vi "Target.vi"() -> ()   [LabVIEW 2013]
uses:
  <vilib>/Platform/TimedLoop/XDataNode/XDataNode.xnode
  <vilib>/Platform/TimedLoop/XDataNode/nitl_modes.ctl
  <vilib>/Platform/TimedLoop/XDataNode/XDNodeRunTimeDep.lvlib
  <vilib>/Platform/TimedLoop/XDataNode/wakeup.ctl
  <vilib>/Platform/TimedLoop/XDataNode/timing_clust.ctl
  <vilib>/rvi/DataTransferAndStorage/Container/XNode/niFpgaContainer.xnode
  <vilib>/rvi/Memory/Memory_Emulation/niFpgaMemoryFastEmulationDramWriteAndRequestData.vi
  <vilib>/rvi/Memory/Memory_Emulation/niFpgaMemoryEmulationDramWriteAndRequestData.vi
  <vilib>/rvi/Memory/Memory_Emulation/niFpgaMemoryEmulationDramRetrieveData.vi
  <vilib>/rvi/interface/RandomDataEmulation/nirviRandomDataFpgaReadWriteTemplate.vi
panel:
  out "I":i32
  out "D-0 2":u16
  out "Addr":u32
  in  "Непрерывно":bool
  out "Number of Elements to Write":u32
  in  "Чтение FIFO":bool
  out "Data":u16
  in  "Input Valid":bool=TRUE
  in  "Address":u32
  in  "Чтение DRAM":bool
  in  "Начальный адрес":u32
  in  "HOST":bool
  in  "D-0":u16
  in  "Запись в DRAM":bool
  in  "Стоп":bool
  in  "Requested Number of Elements":u32=1073152
  in  "2/2":i16=40
  in  "1/2":i16=20
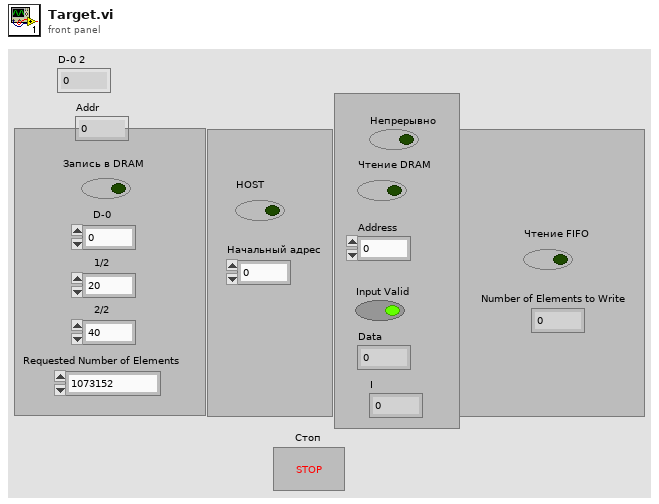
[diagram p1: front panel]
types:
  T1 = typedef "XDNodeRunTimeDep.lvlib/timing_clust.ctl" = cluster{"Expected End [f-1]":u64, "Actual End [f-1]":u64, "Finished Late? [f-1]":bool, "Expected End [i-1]":u64, "Actual End [i-1]":u64, "Finished Late? [i-1]":bool, "Expected Start [i]":u64, "Actual Start [i]":u64, "Expected Start [f]":u64, "Actual Start [f]":u64, "Source Name":string, "Structure Name":string, "Period":i64, "Deadline":i64, "Offset":i64, "Start":i64, "Priority":i32, "Timeout":i32, "Mode":T2, "Wakeup Reason":T3, "Error":errorcluster, "Source Type":string, "Secondary Source Type":string, "Global End Time":u64, "Global Start Time":u64, "Frame Duration":u64, "Iteration Duration":u64, "Assigned CPU":i32, "I/O Scan Engine Mode":u32}
  T2 = typedef "XDNodeRunTimeDep.lvlib/nitl_modes.ctl" = enum32{"No Change", "Process missed periods, maintain original phase", "Discard missed periods, maintain original phase", "Process missed periods, ignore original phase", "Discard missed periods, ignore original phase"}
  T3 = typedef "XDNodeRunTimeDep.lvlib/wakeup.ctl" = enum32{"Normal", "Aborted", "Asynchronous wakeup", "Timing source error", "Timed loop error", "Timeout"}
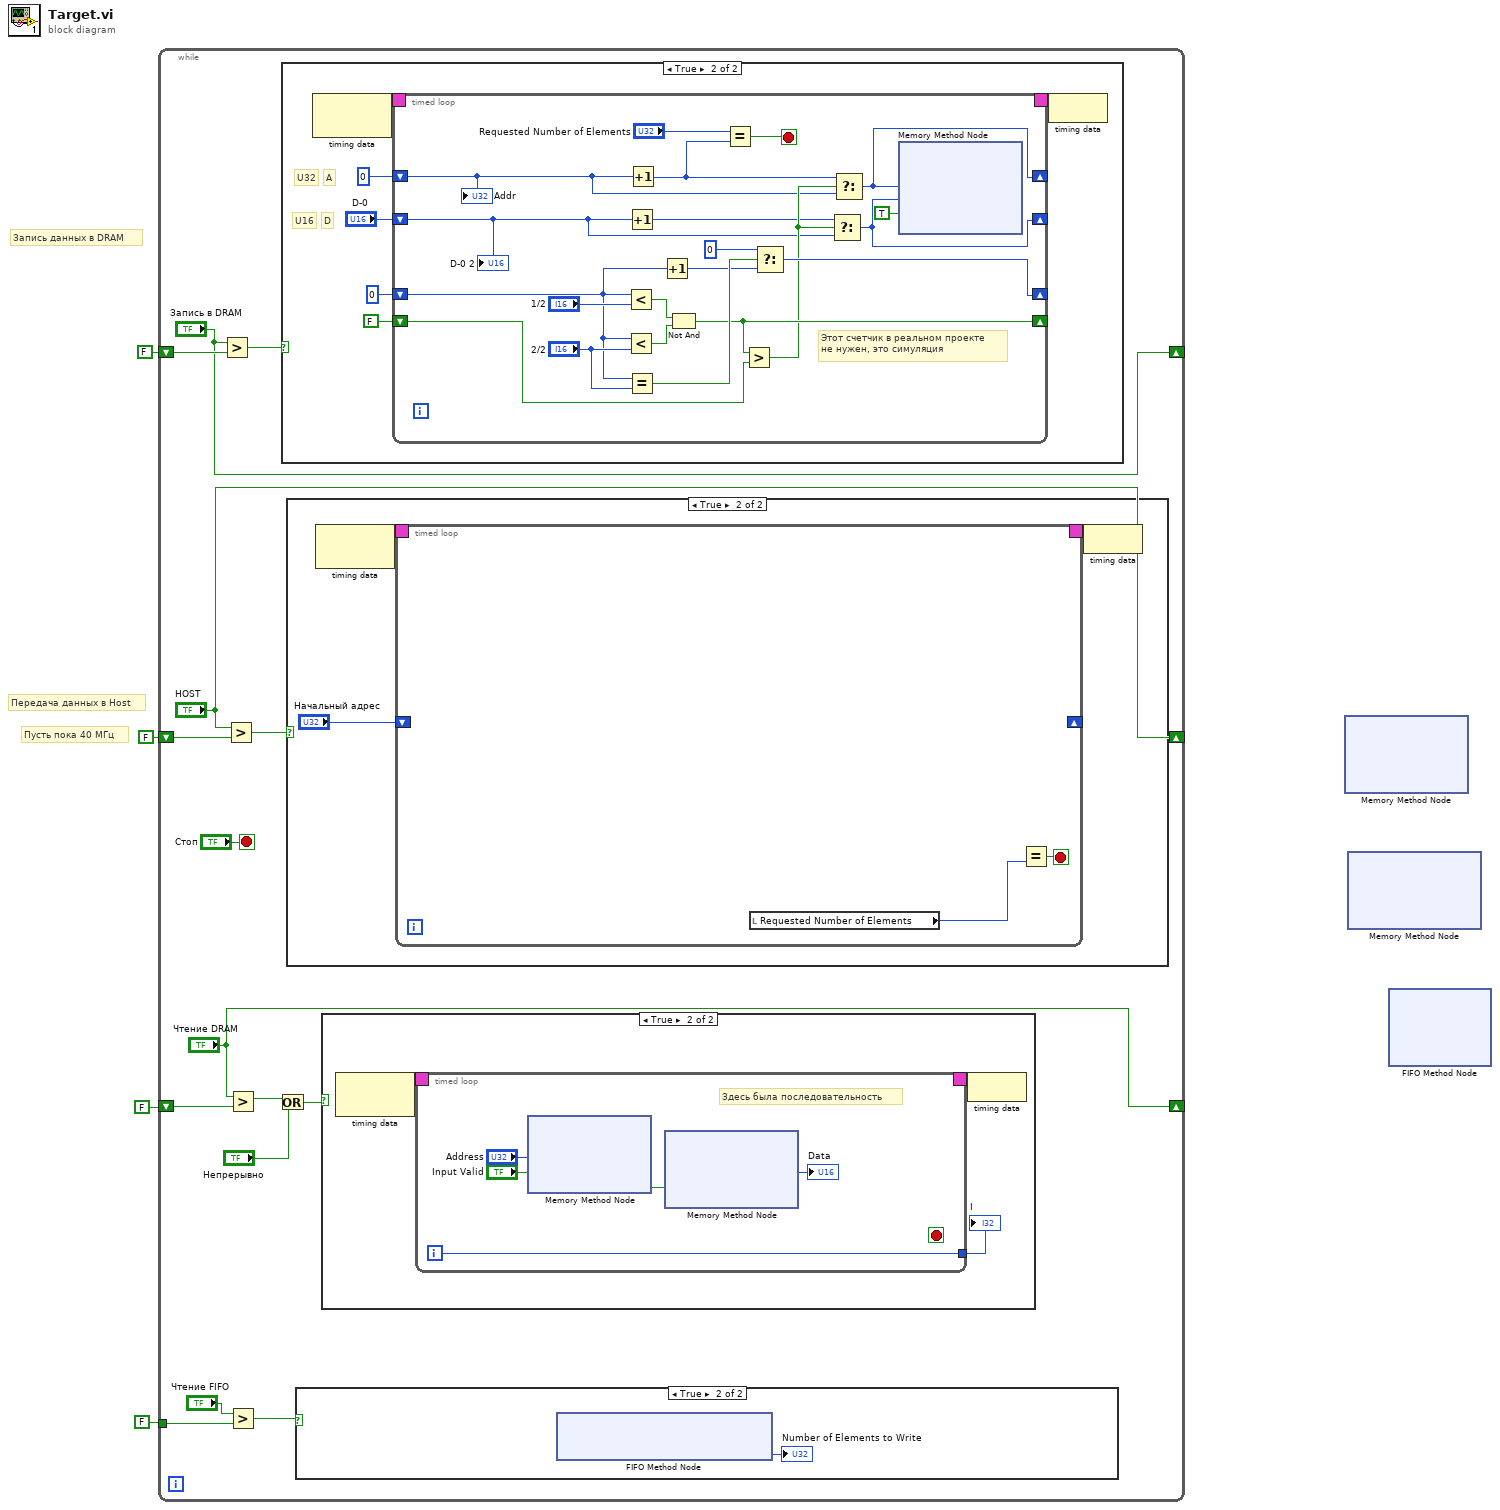
[diagram p0: block diagram]
diagram:
  # "Пусть пока 40 МГц"
  # "Передача данных в Host"
  # "Запись данных в DRAM"
  n1 = while {
    shift-right: ["Запись в DRAM"] -> _
    shift-left: FALSE -> [w18]
    shift-right: ["HOST"] -> _
    shift-left: FALSE -> [w14]
    shift-right: ["Чтение DRAM"] -> _
    shift-left: FALSE -> [w12]
    tunnel: FALSE -> [w9]
    stop <- "Стоп" stop-if-true
    n2 = Greater?(x="Запись в DRAM", y=w18) -> (0:w16:bool)
    n3 = Greater?(x="HOST", y=w14) -> (0:w15:bool)
    n4 = Greater?(x="Чтение DRAM", y=w12) -> (0:w6:bool)
    n5 = Greater?(x="Чтение FIFO", y=w9) -> (0:w8:bool)
    n6 = Or(x=w6, y="Непрерывно") -> (x .or. y?=w7:bool)
    n7 = case shown="True" w16 {
      frame False {
      }
      frame True {
        # "D"
        # "A"
        # "U32"
        # "U16"
        n8 = node-c288() -> (w47:T1)  [unwired: 1 in]
        n9 = timed-loop {
          timing: w47 -> [_]
          timing-out: [_] -> w46
          shift-right: [w60] -> _
          shift-left: i16 0 -> [w62]
          shift-right: [w59] -> _
          shift-left: FALSE -> [w58]
          shift-right: [w50] -> _
          shift-left: "D-0" -> [w56]
          shift-right: [w51] -> _
          shift-left: u32 0 -> [w52]
          stop <- w53 stop-if-true
          # "Этот счетчик в реальном проекте\nне нужен, это симуляция"
          n10 = Less?(x=w62, y="1/2") -> (x < y?=w66:bool)
          n11 = Less?(x=w62, y="2/2") -> (x < y?=w67:bool)
          n12 = Increment(x=w56) -> (x+1=w55:u16)
          n13 = Equal?(x=w62, y="2/2") -> (x = y?=w64:bool)
          n14 = Increment(x=w52) -> (x+1=w49:u32)
          n15 = Increment(x=w62) -> (x+1=w61:i16)
          n16 = Not And(1:w67, 2:w66) -> (0:w59:bool)
          n17 = Equal?(x="Requested Number of Elements", y=w49) -> (x = y?=w53:bool)
          n18 = Greater?(x=w59, y=w58) -> (0:w57:bool)
          n19 = Select(t=i16 0, s=w64, f=w61) -> (s? t:f=w60:i16)
          n20 = Select(t=w55, s=w57, f=w56) -> (s? t:f=w50:u16)
          n21 = Select(t=w49, s=w57, f=w52) -> (s? t:f=w51:u32)
          n22 = xnode ("Memory Method Node")("Address"=w51, "Data"=w50, "Input Valid"=TRUE) -> ()  [unwired: 1 in, 2 out]
          "Addr" <- w52
          "D-0 2" <- w56
        }
        n23 = node-c288(w46) -> ()
      }
    }
    n24 = case shown="True" w15 {
      frame False {
      }
      frame True {
        n25 = node-c288() -> (w34:T1)  [unwired: 1 in]
        n26 = timed-loop {
          shift-right: _ -> [_]
          shift-left: "Начальный адрес" -> [_]
          timing: w34 -> [_]
          timing-out: [_] -> w33
          stop <- w36 stop-if-true
          n27 = local read "Requested Number of Elements"() -> (w37:u32)
          n28 = Equal?(y=w37) -> (x = y?=w36:bool)  [unwired: 1 in]
        }
        n29 = node-c288(w33) -> ()
      }
    }
    n30 = case shown="True" w8 {
      frame False {
      }
      frame True {
        n31 = xnode ("FIFO Method Node")() -> ("Number of Elements to Write"=→"Number of Elements to Write":u32)  [unwired: 1 in, 1 out]
      }
    }
    n32 = case shown="True" w7 {
      frame False {
      }
      frame True {
        n33 = node-c288() -> (w23:T1)  [unwired: 1 in]
        n34 = timed-loop {
          timing: w23 -> [_]
          timing-out: [_] -> w22
          tunnel: [w24] -> w21
          i -> [w24]
          stop <- _ stop-if-true
          # "Здесь была последовательность"
          n35 = xnode ("Memory Method Node")("Address"="Address", "Input Valid"="Input Valid") -> ("Ready For Input"=w26:bool)  [unwired: 1 in, 1 out]
          n36 = xnode ("Memory Method Node")("Ready For Output"=w26) -> ("Data"=→"Data":u16)  [unwired: 1 in, 2 out]
        }
        "I" <- w21
        n37 = node-c288(w22) -> ()
      }
    }
  }
  n38 = xnode ("Memory Method Node")() -> ()  [unwired: 3 in, 2 out]
  n39 = xnode ("Memory Method Node")() -> ()  [unwired: 2 in, 3 out]
  n40 = xnode ("FIFO Method Node")() -> ()  [unwired: 3 in, 2 out]
